vi "SettingsView.vi"(8 "error in (no error)":errorcluster, 11 "Settings.lvclass":refnum<class "Settings.lvclass">) -> (0 "error out":errorcluster, 3 "Settings out":refnum<class "Settings.lvclass">)   [LabVIEW 2016, in "Settings.lvclass"]
uses:
  Settings.lvclass
  Settings.lvclass/Settings.ctl
panel:
  in  "Port":u16=50000
  in  "IP":string="140.252.32.223"
  in  "OK Button":bool
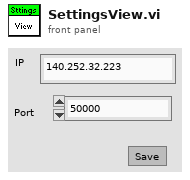
[diagram p1: front panel]
types:
  T1 = enum32{"Invalid", "Standard", "Closed", "Hidden", "Minimized", "Maximized"}
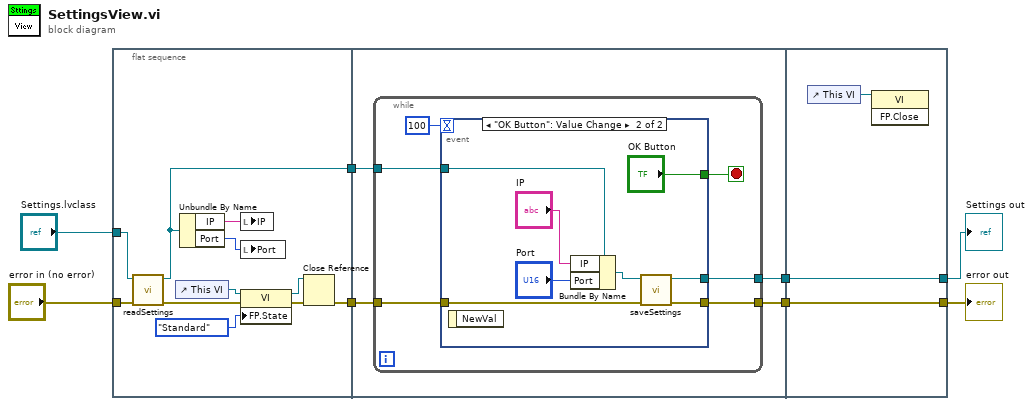
[diagram p0: block diagram]
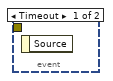
[diagram p2: hidden frame]
diagram:
  n1 = flat-sequence {
    tunnel: "Settings.lvclass" -> [w19]
    tunnel: [w16] -> w7
    tunnel: "error in (no error)" -> [w15]
    tunnel: [w10] -> w5
    tunnel: w7 -> [w23]
    tunnel: w5 -> [w22]
    tunnel: [w21] -> w4
    tunnel: [w20] -> w3
    tunnel: [w39] -> w1
    tunnel: w4 -> [w39]
    tunnel: [w38] -> w2
    tunnel: w3 -> [w38]
    frame #0 {
      n2 = call "readSettings.vi"("error in (no error)"=w15, "Settings in"=w19) -> ("error out"=w12:errorcluster, "Settings out"=w16:refnum<class "Settings.lvclass">)  [unwired: 8 in]
      n3 = control-ref of="This VI"() -> (w14:refnum<vi>)
      n4 = Unbundle By Name(w16) -> ("IP"=w18:string, "Port"=w17:u16)
      n5 = local write "IP"(w18) -> ()
      n6 = local write "Port"(w17) -> ()
      n7 = property class="VI"(reference=w14, error in=w12, "FP.State"=T1."Standard" ("Front Panel Window:State")) -> (reference out=w9:refnum<vi>, error out=w11:errorcluster)
      n8 = Close Reference(reference=w9, error in (no error)=w11) -> (error out=w10:errorcluster)
    }
    frame #1 {
      n9 = while {
        tunnel: w23 -> [w27]
        tunnel: w22 -> [w26]
        tunnel: [w25] -> w21
        tunnel: [w24] -> w20
        stop <- w28 stop-if-true
        n10 = event shown="[1] \"OK Button\": Value Change" {
          selector: _ -> [_ _]
          dyn-events: _ -> [_ _]
          timeout: 100 -> [_ _]
          tunnel: [_ "OK Button"] -> w28
          tunnel: w27 -> [_ w36]
          tunnel: w26 -> [_ w32]
          tunnel: [_ w31] -> w25
          tunnel: [_ w30] -> w24
          event Timeout {
            n11 = event-data() -> ()  [unwired: 1 in, 1 out]
          }
          event "OK Button": Value Change {
            n12 = event-data() -> ()  [unwired: 1 in, 1 out]
            n13 = Bundle By Name(cluster=w36, "IP"="IP", "Port"="Port") -> (w33:refnum<class "Settings.lvclass">)
            n14 = call "saveSettings.vi"("error in (no error)"=w32, "Settings in"=w33) -> ("error out"=w30:errorcluster, "Settings out"=w31:refnum<class "Settings.lvclass">)  [unwired: 8 in]
          }
        }
      }
    }
    frame #2 {
      n15 = control-ref of="This VI"() -> (w40:refnum<vi>)
      n16 = invoke class="VI" method="FP.Close"(reference=w40) -> ()  [unwired: 2 in, 3 out]
    }
  }
  "error out" <- w2
  "Settings out" <- w1
